vi "RPT_CalibrationInfo.vi"(11 "Test Info":T1) -> (3 "Array":string[][](array[string]))   [LabVIEW 2024]
uses:
  Control Definitions/DEF_TestInfo.ctl
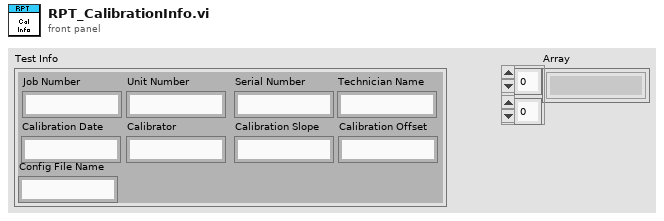
[diagram p1: front panel]
types:
  T1 = typedef "DEF_TestInfo.ctl" = cluster{"Job Number":string, "Unit Number":string, "Serial Number":string, "Technician Name":string, "Calibration Date":string, "Calibrator":string, "Calibration Slope":string, "Calibration Offset":string, "Config File Name":string}
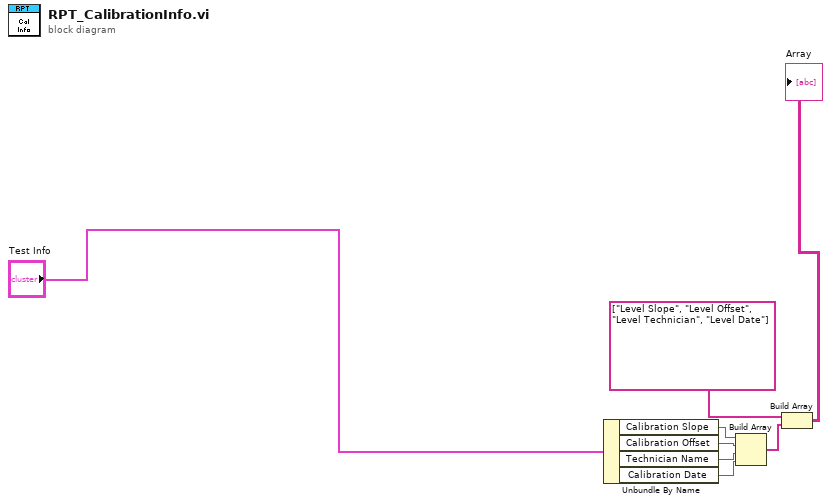
[diagram p0: block diagram]
diagram:
  n1 = Unbundle By Name("Test Info") -> ("Calibration Slope"=w2:string, "Calibration Offset"=w3:string, "Technician Name"=w4:string, "Calibration Date"=w5:string)
  n2 = Build Array(w2, w3, w4, w5) -> (w6:string[])
  n3 = Build Array(string[] ["Level Slope", "Level Offset", "Level Technician", "Level Date"] ("appended array"), w6) -> (→"Array":string[][])
